vi "Time.Tamper Check.vi"(8 "error in (no error)":errorcluster, 11 "Path":path) -> (0 "error out":errorcluster, 1 "File Save Error":errorcluster, 3 "Time OK":bool)   [LabVIEW 2019]
uses:
  <vilib>/Utility/sysdir.llb/System Directory Type.ctl
  <vilib>/KATE/Files/File Utils.lvlib
panel:
  out "Delta Time":dbl format="%#.12g"
  out "Current Time":dbl format="%#.12g"
  out "Saved Time":dbl format="%#.12g"
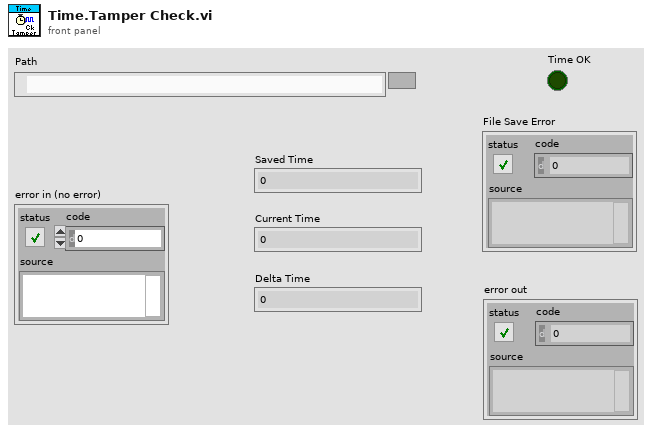
[diagram p1: front panel]
types:
  T1 = enum16{"open", "replace", "create", "open or create", "replace or create", "replace or create with confirmation"}
  T2 = typedef "System Directory Type.ctl" = i32
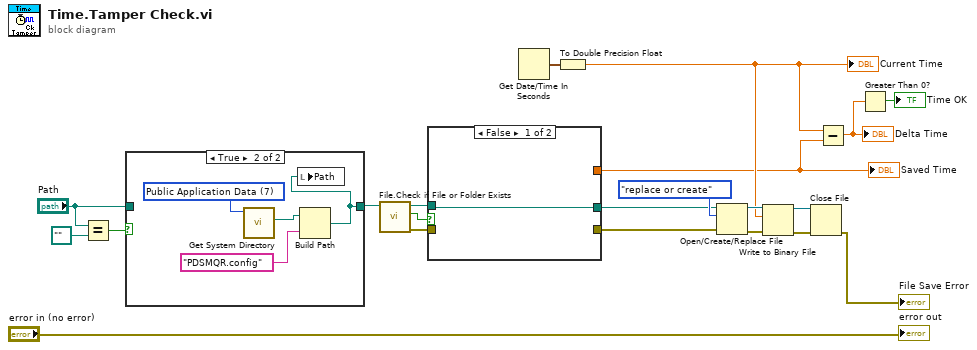
[diagram p0: block diagram]
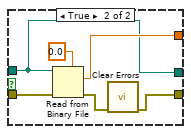
[diagram p3: hidden frame]
diagram:
  n1 = Equal?(x="Path", y=path "") -> (x = y?=w6:bool)
  n2 = case shown="True" w6 {
    tunnel: "Path" -> [w22 _]
    tunnel: [w22 w23] -> w4
    frame False {
    }
    frame True {
      w26 = T2 7 items=["User Home"=0, "User Desktop"=1, "User Documents"=2, "User Application Data"=3, "User Preferences"=4, "User Temporary"=5, "Public Documents"=6, "Public Application Data"=7, "Public Preferences"=8, "Public Cache"=13, "System Core Libraries"=9, "System Installed Libraries"=10, "Application Files"=11, "Boot Volume Root"=12] ("system directory type")
      n3 = call <vilib>:"Get System Directory.vi"("system directory type"=w26) -> ("system directory"=w25:path)  [unwired: 10 in]
      n4 = Build Path(base path=w25, name or relative path="PDSMQR.config") -> (appended path=w23:path)
      n5 = local write "Path"(w23) -> ()
    }
  }
  n6 = call <vilib>:"File.Check if File or Folder Exists.vi"("Path"=w4) -> ("error out"=w19:errorcluster, "Exists"=w21:bool, "Dup Path"=w20:path)  [unwired: 6 in, 2 out]
  n7 = case shown="False" w21 {
    tunnel: w20 -> [w27 w28]
    tunnel: w19 -> [_ w33]
    tunnel: [_ w31] -> w10
    tunnel: [_ w29] -> w12
    tunnel: [w27 w28] -> w1
    frame False {
    }
    frame True {
      n8 = Read from Binary File(5:0.0, 8:w33, 11:w28) -> (0:w30:errorcluster, 2:w31:dbl)  [unwired: 3 in, 2 out]
      n9 = call <vilib>:"Clear Errors.vi"("error in (no error)"=w30) -> ("error out"=w29:errorcluster)  [unwired: 5 in, 1 out]
    }
  }
  "Saved Time" <- w10
  n10 = Get Date/Time In Seconds() -> (seconds since 1Jan1904=w18:timestamp)
  n11 = To Double Precision Float(number=w18) -> (double precision float=w11:dbl)
  "Current Time" <- w11
  n12 = Open/Create/Replace File(file path (use dialog)=w1, error in=w12, operation (0:open)=T1."replace or create") -> (refnum out=w14:refnum<file>, error out=w17:errorcluster)  [unwired: 3 in, 1 out]
  n13 = Write to Binary File(file (use dialog)=w14, data=w11, error in=w17) -> (refnum out=w13:refnum<file>, error out=w16:errorcluster)  [unwired: 3 in, 1 out]
  n14 = Close File(refnum=w13, error in=w16) -> (error out=→"File Save Error":errorcluster)  [unwired: 1 out]
  n15 = Subtract(x=w11, y=w10) -> (x-y=w8:dbl)
  "Delta Time" <- w8
  n16 = Greater Than 0?(x=w8) -> (x > 0?=→"Time OK":bool)
  "error out" <- "error in (no error)"
